vi "Test Variant to Array of Variants.vi"() -> ()   [LabVIEW 2019, in "Control Experiment.lvclass"]
uses:
  Control Experiment.lvclass
panel:
  out "Variant (1D array)":variant[][](array[variant])
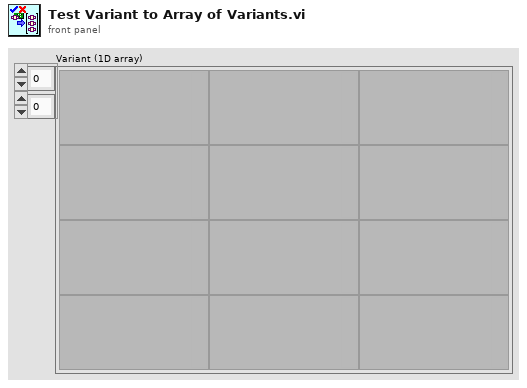
[diagram p1: front panel]
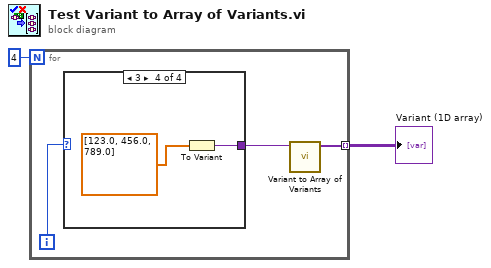
[diagram p0: block diagram]
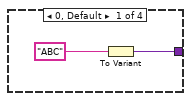
[diagram p2: hidden frame]
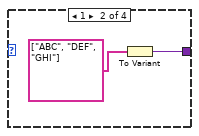
[diagram p3: hidden frame]
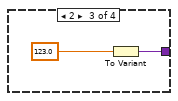
[diagram p4: hidden frame]
diagram:
  n1 = for {
    N: 4 -> [_]
    tunnel: [w5] -> w2 mode=indexing
    i -> [w4]
    n2 = case shown="3" w4 {
      tunnel: [w6 w8 w11 w13] -> w3
      frame 0, Default {
        n3 = To Variant(anything="ABC" ("String")) -> (Variant=w6:variant)
      }
      frame 1 {
        n4 = To Variant(anything=string[] ["ABC", "DEF", "GHI"] ("Array")) -> (Variant=w8:variant)
      }
      frame 2 {
        n5 = To Variant(anything=123.0) -> (Variant=w11:variant)
      }
      frame 3 {
        n6 = To Variant(anything=dbl[] [123.0, 456.0, 789.0]) -> (Variant=w13:variant)
      }
    }
    n7 = call "Variant to Array of Variants.vi"("value"=w3) -> ("Variant (1D array)"=w5:variant[])  [unwired: 9 in, 1 out]
  }
  "Variant (1D array)" <- w2
